vi "Rotations (SubVI).vi"(0 "RelayValue":T1=enum."Forward", 1 "SwitchValue":bool, 2 "Reset":bool) -> (10 "Rotations":i32)   [LabVIEW 2013]
uses:
  <vilib>/Rock Robotics/WPI/Relay/WPI_RelayValue.ctl
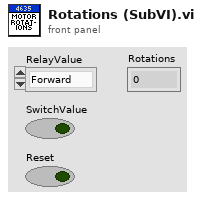
[diagram p1: front panel]
types:
  T1 = typedef "WPI_RelayValue.ctl" = enum16{"Off", "On", "Forward", "Reverse"}
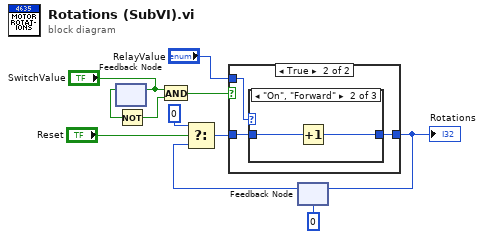
[diagram p0: block diagram]
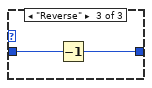
[diagram p4: hidden frame]
diagram:
  n1 = feedback #1() -> (w3:bool)  [unwired: 1 in]
  n2 = feedback-in #1("SwitchValue") -> ()
  n3 = Not(x=w3) -> (.not. x?=w4:bool)
  n4 = And(x="SwitchValue", y=w4) -> (x .and. y?=w9:bool)
  n5 = feedback #2(0) -> (w8:i32)
  n6 = Select(t=0, s="Reset", f=w8) -> (s? t:f=w10:i32)
  n7 = case shown="True" w9 {
    tunnel: w10 -> [w12 w14]
    tunnel: [w12 w13] -> w11
    tunnel: "RelayValue" -> [_ w15]
    frame False {
    }
    frame True {
      n8 = case shown="\"On\", \"Forward\"" w15 {
        tunnel: w14 -> [w16 w18 w20]
        tunnel: [w16 w17 w19] -> w13
        frame "Off", Default {
        }
        frame "On", "Forward" {
          n9 = Increment(x=w18) -> (x+1=w17:i32)
        }
        frame "Reverse" {
          n10 = Decrement(x=w20) -> (x-1=w19:i32)
        }
      }
    }
  }
  "Rotations" <- w11
  n11 = feedback-in #2(w11) -> ()
